vi "niRFSysCalReader Fetch Measurement Offset.vi"(6 "Search Settings":T1={"Priority"=enum."Reference Level", "Ref Level  Tolerance (dB)"=1.0, "Frequency Tolerance (Hz)"=10000000.0} {"Frequency Tolerance (Hz)" format="%#_6p"}, 8 "error in":errorcluster, 9 "Actual Reference Level (dBm)":dbl, 10 "Actual Frequency (Hz)":dbl format="%#_6p", 11 "niRFSysCalReader Handle":T3) -> (0 "error out":errorcluster, 1 "Equivalent Calibration State":T2={"Frequency (Hz)"=nan, "Ref Level (dBm)"=nan, "Ext. Gain (dB)"=nan, "Cal Error (dB)"=nan} {"Cal Error (dB)" format="%#_6p"; "Frequency (Hz)" format="%#_6p"; "Ref Level (dBm)" format="%#_6p"; "Ext. Gain (dB)" format="%#_6p"}, 2 "Measurement Offset (dB)":dbl=nan, 3 "niRFSysCalReader Handle out":T3)   [LabVIEW 2016, in "niRFSysCalReader.lvlib"]
doc: "Returns the recommended measurement offset. This value should be added to power results. \n\n<b>Note:</b> Measurement offset is an <b>alternative</b> to receiver offset. The measurement offset is selected by choosing the path loss from the system calibration data, where the receiver's current settings best matches a system calibration setting. It may be advantageous to apply a measurement offset, instead of a receiver offset, if changes to a receiver's actual reference level has unintended affects on non-power related measurements, e.g. Error Vector Magntiude (EVM), that are performed on the same acquisition that is used for the power measurement.\n\n<b>Actual Reference Level</b> = Receiver Reference Level + Receiver External Gain Setting"
uses:
  niRFSysCalReader.lvlib
  INCLUDES/niRFSysCalReader Handle.ctl
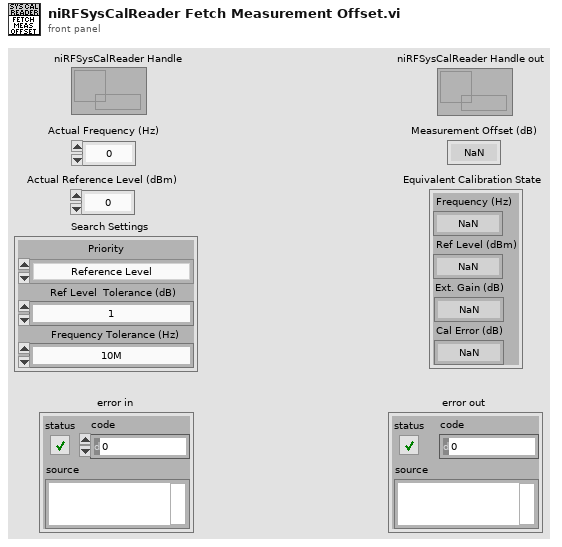
[diagram p1: front panel]
types:
  T1 = cluster{"Priority":enum16{"Frequency", "Reference Level"}, "Ref Level  Tolerance (dB)":dbl, "Frequency Tolerance (Hz)":dbl}
  T2 = cluster{"Frequency (Hz)":dbl, "Ref Level (dBm)":dbl, "Ext. Gain (dB)":dbl, "Cal Error (dB)":dbl}
  T3 = typedef "niRFSysCalReader.lvlib/niRFSysCalReader Handle.ctl" = refnum<data-value>
  T4 = cluster{dbl[], dbl[], cluster{"Frequency (Hz)":dbl, "Power (dBm)":dbl, "Receiver Offset (dB)":dbl, "Error (dB)":dbl}[]}
  T5 = cluster{"Frequency (Hz)":dbl, "Power (dBm)":dbl}[]
  T6 = cluster{"Frequency (Hz)":dbl, "Power (dBm)":dbl, "Receiver Offset (dB)":dbl, "Error (dB)":dbl}
  T7 = cluster{"Search Priority":enum16{"Frequency", "Reference Level"}, "Ref Level Search Tolerance (dB)":dbl, "Frequency Search Tolerance (Hz)":dbl}
  T8 = cluster{"Ref Level Search Tolerance (dB)":dbl, "Frequency Search Tolerance (Hz)":dbl, cluster{"Frequency (Hz)":dbl, "Power (dBm)":dbl, "Receiver Offset (dB)":dbl, "Error (dB)":dbl}}[]
  T9 = cluster{"Frequency (Hz)":dbl, "Power (dBm)":dbl, "Receiver Offset (dB)":dbl, "Error (dB)":dbl}[]
  T10 = cluster{"Frequency Tolerance (Hz)":dbl, "Ref Level  Tolerance (dB)":dbl, cluster{"Frequency (Hz)":dbl, "Power (dBm)":dbl, "Receiver Offset (dB)":dbl, "Error (dB)":dbl}}[]
  T11 = cluster{"Ref Level  Tolerance (dB)":dbl, "Frequency Tolerance (Hz)":dbl, cluster{"Frequency (Hz)":dbl, "Power (dBm)":dbl, "Receiver Offset (dB)":dbl, "Error (dB)":dbl}}[]
  T12 = cluster{bool, bool, cluster{"Frequency (Hz)":bool, "Power (dBm)":bool, "Receiver Offset (dB)":bool, "Error (dB)":bool}}
  T13 = cluster{dbl, dbl, cluster{"Frequency (Hz)":dbl, "Power (dBm)":dbl, "Receiver Offset (dB)":dbl, "Error (dB)":dbl}}[]
  T14 = cluster{bool, bool, cluster{"Frequency (Hz)":bool, "Power (dBm)":bool, "Receiver Offset (dB)":bool, "Error (dB)":bool}}[]
  T15 = cluster{dbl, dbl, cluster{"Frequency (Hz)":dbl, "Power (dBm)":dbl, "Receiver Offset (dB)":dbl, "Error (dB)":dbl}}
  T16 = cluster{"Frequency (Hz)":dbl, "Power (dBm)":dbl, dbl, "Error (dB)":dbl}
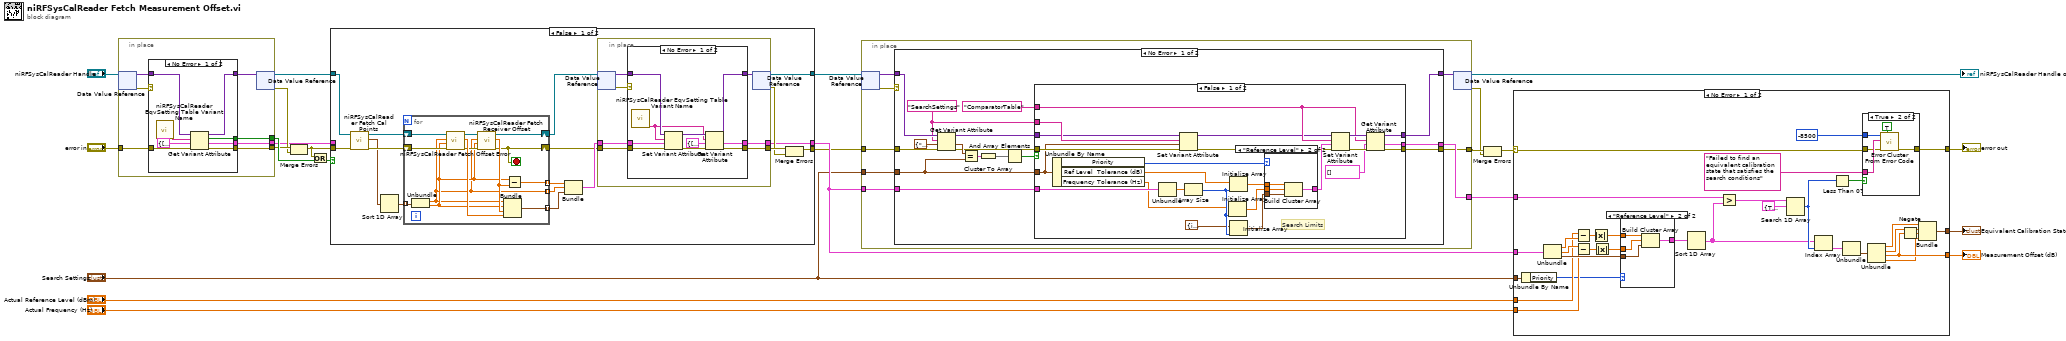
[diagram p0: block diagram]
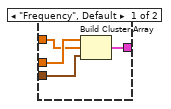
[diagram p2: hidden frame]
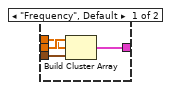
[diagram p5: hidden frame]
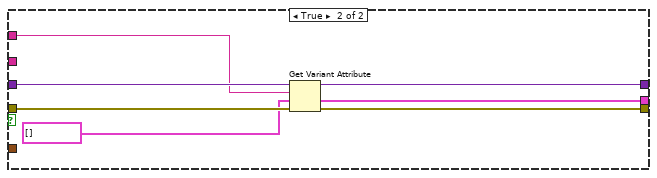
[diagram p6: hidden frame]
diagram:
  n1 = in-place {
    in-place-border: [w28] -> w19
    in-place-border: [w27] -> w22
    in-place-border: [w26] -> w15
    in-place-border: "error in" -> [w24]
    n2 = in-place-dvr #1("niRFSysCalReader Handle") -> (w30:variant, w25:errorcluster)
    n3 = case shown="No Error" w25 {
      tunnel: w30 -> [w38 w40]
      tunnel: [w36 w40] -> w29
      tunnel: [w35 w39] -> w28
      tunnel: [w34 _] -> w27
      tunnel: [w33 _] -> w26
      tunnel: w24 -> [w31 w39]
      frame No Error {
        n4 = call "niRFSysCalReader EqvSetting Table Variant Name.vi"() -> ("Equivalent Setting Table Name"=w32:string)  [unwired: 11 in]
        n5 = Get Variant Attribute(Variant=w38, name=w32, default value (empty Variant)=T4 {[], [], []} ("output cluster"), error in=w31) -> (duplicate Variant=w36:variant, found=w34:bool, value=w33:T4, error out=w35:errorcluster)
      }
      frame Error {
      }
    }
    n6 = in-place-dvr #1(w29) -> (w21:T3, w18:errorcluster)
  }
  n7 = Merge Errors(w19, w18) -> (w13:errorcluster)
  n8 = Or(x=w13, y=w22) -> (x .or. y?=w14:bool)
  n9 = case shown="False" w14 {
    tunnel: w21 -> [w50 w93]
    tunnel: w13 -> [w46 w91]
    tunnel: [w43 w93] -> w10
    tunnel: [w42 w92] -> w7
    tunnel: w15 -> [_ w92]
    tunnel: [w41 w91] -> w6
    frame False {
      n10 = call "niRFSysCalReader Fetch Cal Points.vi"("error in"=w46, "niRFSysCalReader Handle"=w50) -> ("error out"=w56:errorcluster, "Cal Points"=w55:T5, "niRFSysCalReader Handle out"=w57:T3)  [unwired: 7 in]
      n11 = Sort 1D Array(array=w55) -> (sorted array=w52:T5)
      n12 = for {
        shift-right: [w83] -> w49
        shift-left: w57 -> [w87]
        shift-right: [w78] -> w47
        shift-left: w56 -> [w86]
        tunnel: w52 -> [w90] mode=indexing
        tunnel: [w88] -> w51 mode=indexing
        tunnel: [w80] -> w54 mode=indexing
        tunnel: [w79] -> w53 mode=indexing
        stop <- w78 stop-if-true
        n13 = Unbundle(w90) -> ("Frequency (Hz)"=w79:dbl, "Power (dBm)"=w81:dbl)
        n14 = call "niRFSysCalReader Fetch Offset Error.vi"("error in"=w86, "Level (dBm)"=w81, "Frequency (Hz)"=w79, "niRFSysCalReader Handle"=w87) -> ("error out"=w84:errorcluster, "Error (dB)"=w89:dbl, "niRFSysCalReader Handle out"=w85:T3)  [unwired: 5 in]
        n15 = call "niRFSysCalReader Fetch Receiver Offset.vi"("error in"=w84, "Reference Level (dBm)"=w81, "Frequency (Hz)"=w79, "niRFSysCalReader Handle"=w85) -> ("error out"=w78:errorcluster, "Receiver Offset (dB)"=w82:dbl, "niRFSysCalReader Handle out"=w83:T3)  [unwired: 5 in]
        n16 = Bundle("Frequency (Hz)"=w79, "Power (dBm)"=w81, "Receiver Offset (dB)"=w82, "Error (dB)"=w89) -> (w88:T6)  [unwired: 1 in]
        n17 = Subtract(x=w81, y=w82) -> (x-y=w80:dbl)
      }
      n18 = Bundle(w54, w53, w51) -> (w48:T4)  [unwired: 1 in]
      n19 = in-place {
        in-place-border: [w62] -> w45
        in-place-border: [w61] -> w42
        in-place-border: w48 -> [w60]
        in-place-border: w47 -> [w58]
        n20 = in-place-dvr #2(w49) -> (w64:variant, w59:errorcluster)
        n21 = case shown="No Error" w59 {
          tunnel: w64 -> [w69 w77]
          tunnel: [w74 w77] -> w63
          tunnel: [w73 w75] -> w62
          tunnel: [w72 w76] -> w61
          tunnel: w60 -> [w67 w76]
          tunnel: w58 -> [w71 w75]
          frame No Error {
            n22 = call "niRFSysCalReader EqvSetting Table Variant Name.vi"() -> ("Equivalent Setting Table Name"=w65:string)  [unwired: 11 in]
            n23 = Set Variant Attribute(Variant=w69, name=w65, value=w67, error in=w71) -> (Variant out=w68:variant, error out=w70:errorcluster)  [unwired: 1 out]
            n24 = Get Variant Attribute(Variant=w68, name=w65, default value (empty Variant)=T4 {[], [], []}, error in=w70) -> (duplicate Variant=w74:variant, value=w72:T4, error out=w73:errorcluster)  [unwired: 1 out]
          }
          frame Error {
          }
        }
        n25 = in-place-dvr #2(w63) -> (w43:T3, w44:errorcluster)
      }
      n26 = Merge Errors(w45, w44) -> (w41:errorcluster)
    }
    frame True {
    }
  }
  n27 = in-place {
    in-place-border: "Search Settings" -> [w98]
    in-place-border: [w97] -> w8
    in-place-border: w7 -> [w96]
    in-place-border: w6 -> [w95]
    in-place-border: [w94] -> w4
    n28 = in-place-dvr #3(w10) -> (w100:variant, w101:errorcluster)
    n29 = case shown="No Error" w101 {
      tunnel: w100 -> [w117 w158]
      tunnel: [w111 w158] -> w99
      tunnel: w98 -> [w102 _]
      tunnel: [w107 _] -> w97
      tunnel: w96 -> [w106 _]
      tunnel: [w105 w157] -> w94
      tunnel: w95 -> [w104 w157]
      frame No Error {
        w103 = "SearchSettings" ("name")
        n30 = Get Variant Attribute(Variant=w117, name=w103, default value (empty Variant)=T7 {"Search Priority"=enum."Frequency", "Ref Level Search Tolerance (dB)"=-inf, "Frequency Search Tolerance (Hz)"=-inf} ("output cluster"), error in=w104) -> (duplicate Variant=w112:variant, value=w116:T7, error out=w113:errorcluster)  [unwired: 1 out]
        n31 = Equal?(x=w116, y=w102) -> (x = y?=w114:cluster{bool, bool, bool})
        n32 = Cluster To Array(cluster=w114) -> (array=w108:bool[])
        n33 = And Array Elements(Boolean array=w108) -> (logical AND=w109:bool)
        n34 = case shown="False" w109 {
          tunnel: w113 -> [w126 w156]
          tunnel: w112 -> [w124 w155]
          tunnel: [w132 w154] -> w111
          tunnel: "ComparatorTable" ("name") -> [w129 w153]
          tunnel: [w128 w151] -> w107
          tunnel: w102 -> [w121 _]
          tunnel: w106 -> [w134 _]
          tunnel: [w127 w150] -> w105
          tunnel: w103 -> [w125 _]
          frame False {
            # "Search Limits"
            n35 = Unbundle By Name(w121) -> ("Priority"=w120:enum16{"Frequency", "Reference Level"}, "Ref Level  Tolerance (dB)"=w119:dbl, "Frequency Tolerance (Hz)"=w118:dbl)
            n36 = Unbundle(w134) -> (w140:dbl[])  [unwired: 2 out]
            n37 = Set Variant Attribute(Variant=w124, name=w125, value=w121, error in=w126) -> (Variant out=w123:variant, error out=w122:errorcluster)  [unwired: 1 out]
            n38 = Array Size(array=w140) -> (size(s)=w139:i32)
            n39 = Initialize Array(w118, w139) -> (w136:dbl[])
            n40 = Initialize Array(w119, w139) -> (w135:dbl[])
            n41 = Initialize Array(T6 {"Frequency (Hz)"=inf, "Power (dBm)"=inf, "Receiver Offset (dB)"=inf, "Error (dB)"=inf}, w139) -> (w138:T9)
            n42 = case shown="\"Reference Level\"" w120 {
              tunnel: w135 -> [w144 w149]
              tunnel: w136 -> [w145 w148]
              tunnel: [w142 w147] -> w133
              tunnel: w138 -> [w143 w146]
              frame "Frequency", Default {
                n43 = Build Cluster Array(w145, w144, w143) -> (w142:T10)
              }
              frame "Reference Level" {
                n44 = Build Cluster Array(w149, w148, w146) -> (w147:T11)
              }
            }
            n45 = Set Variant Attribute(Variant=w123, name=w129, value=w133, error in=w122) -> (Variant out=w141:variant, error out=w131:errorcluster)  [unwired: 1 out]
            n46 = Get Variant Attribute(Variant=w141, name=w129, default value (empty Variant)=T8 [], error in=w131) -> (duplicate Variant=w132:variant, value=w128:T8, error out=w127:errorcluster)  [unwired: 1 out]
          }
          frame True {
            n47 = Get Variant Attribute(Variant=w155, name=w153, default value (empty Variant)=T8 [], error in=w156) -> (duplicate Variant=w154:variant, value=w151:T8, error out=w150:errorcluster)  [unwired: 1 out]
          }
        }
      }
      frame Error {
      }
    }
    n48 = in-place-dvr #3(w99) -> (→"niRFSysCalReader Handle out":T3, w1:errorcluster)
  }
  n49 = Merge Errors(w4, w1) -> (w2:errorcluster)
  n50 = case shown="No Error" w2 {
    selector: w2 -> [w165 w204]
    tunnel: "Actual Reference Level (dBm)" -> [w176 _]
    tunnel: "Actual Frequency (Hz)" -> [w175 _]
    tunnel: [w169 w204] -> w12
    tunnel: [w168 _] -> w3
    tunnel: [w162 _] -> w11
    tunnel: w8 -> [w167 _]
    tunnel: w7 -> [w166 _]
    tunnel: "Search Settings" -> [w160 _]
    frame No Error {
      n51 = Unbundle By Name(w160) -> ("Priority"=w159:enum16{"Frequency", "Reference Level"})
      n52 = Unbundle(w166) -> (w188:dbl[], w185:dbl[], w178:T9)
      n53 = Subtract(x=w176, y=w188) -> (x-y=w189:dbl[])
      n54 = Subtract(x=w185, y=w175) -> (x-y=w187:dbl[])
      n55 = Absolute Value(x=w189) -> (abs(x)=w180:dbl[])
      n56 = Absolute Value(x=w187) -> (abs(x)=w179:dbl[])
      n57 = case shown="\"Reference Level\"" w159 {
        tunnel: w180 -> [w192 w197]
        tunnel: w179 -> [w193 w196]
        tunnel: w178 -> [w190 w195]
        tunnel: [w191 w194] -> w177
        frame "Frequency", Default {
          n58 = Build Cluster Array(w193, w192, w190) -> (w191:T13)
        }
        frame "Reference Level" {
          n59 = Build Cluster Array(w197, w196, w195) -> (w194:T13)
        }
      }
      n60 = Sort 1D Array(array=w177) -> (sorted array=w163:T13)
      n61 = Greater?(x=w167, y=w163) -> (0:w182:T14)
      n62 = Search 1D Array(1D array=w182, element=T12 {TRUE, TRUE, {"Frequency (Hz)"=TRUE, "Power (dBm)"=TRUE, "Receiver Offset (dB)"=TRUE, "Error (dB)"=TRUE}}) -> (index of element=w164:i32)  [unwired: 1 in]
      n63 = Index Array(array=w163, index=w164) -> (element=w174:T15)
      n64 = Less Than 0?(x=w164) -> (x < 0?=w186:bool)
      n65 = Unbundle(w174) -> (w173:T6)  [unwired: 2 out]
      n66 = case shown="True" w186 {
        tunnel: [w198 w203] -> w169
        tunnel: "Failed to find an equivalent calibration state that satisfies the search conditions" -> [_ w202]
        tunnel: -8500 ("error code (0)") -> [_ w201]
        tunnel: w165 -> [w198 w199]
        frame False {
        }
        frame True {
          n67 = call <vilib>:"Error Cluster From Error Code.vi"("show call chain? (False)"=TRUE, "error in (no error)"=w199, "error message (\"\")"=w202, "error code (0)"=w201) -> ("error out"=w203:errorcluster)  [unwired: 5 in]
        }
      }
      n68 = Unbundle(w173) -> ("Frequency (Hz)"=w172:dbl, "Power (dBm)"=w171:dbl, "Receiver Offset (dB)"=w162:dbl, "Error (dB)"=w161:dbl)
      n69 = Negate(x=w162) -> (-x=w170:dbl)
      n70 = Bundle("Frequency (Hz)"=w172, "Power (dBm)"=w171, w170, "Error (dB)"=w161) -> (w168:T16)  [unwired: 1 in]
    }
    frame Error {
    }
  }
  "error out" <- w12
  "Measurement Offset (dB)" <- w11
  "Equivalent Calibration State" <- w3
